vi "Full_Client_Name.vi"() -> (0 "Client Name":string)   [LabVIEW 2010]
uses:
  Anemometry/Anemometry Sub Vis/Globals/Preference_global.vi
  Anemometry/Anemometry Sub Vis/Globals/Dynamic_call_global.ph.vi
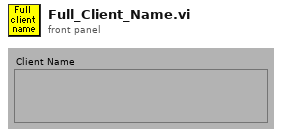
[diagram p1: front panel]
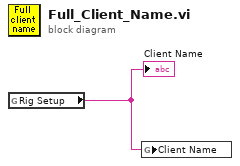
[diagram p0: block diagram]
diagram:
  n1 = global read "Preference_global.vi" "Rig Setup"() -> (w1:string)
  "Client Name" <- w1
  n2 = global write "Dynamic_call_global.ph.vi" "Client Name"(w1) -> ()
